vi "16_2.vi"() -> ()   [LabVIEW 2018]
uses:
  <userlib>/_OpenG.lib/array/array.llb/Sort 1D Array (I32)__ogtk.vi
  <userlib>/_OpenG.lib/array/array.llb/Reorder 1D Array2 (I32)__ogtk.vi
  <userlib>/_OpenG.lib/array/array.llb/Reorder 1D Array2 (Variant)__ogtk.vi
panel:
  out "product":dbl
  out "array":i32[](array[numeric])
  out "Array 6":string[](array[string])
  out "Array 2":cluster{string[]}[](array[cluster])
  out "Array 3":i32[](array[numeric])
  out "your ticket":string
  out "nearby tickets":string[](array[string])
  out "first subarray":string[](array[string])
  in  "Input":string
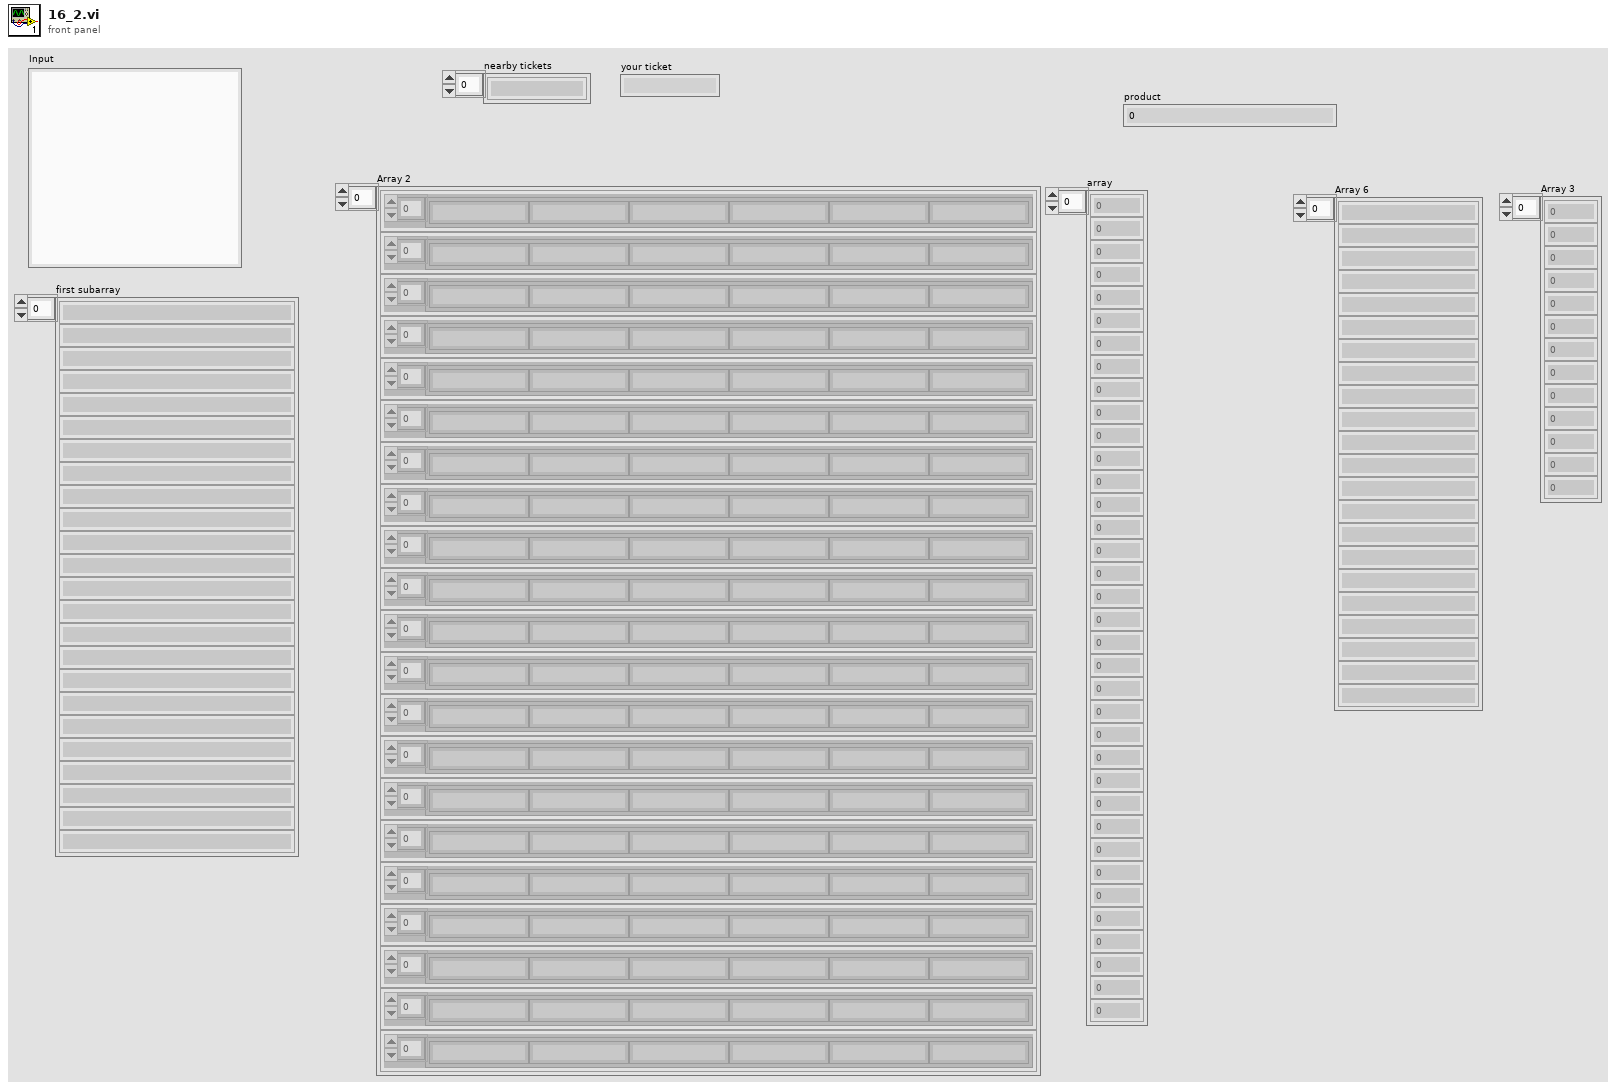
[diagram p1: front panel]
types:
  T1 = cluster{"Min1":i32, "Max1":i32, "Min2":i32, "Max2":i32, "Field":string}
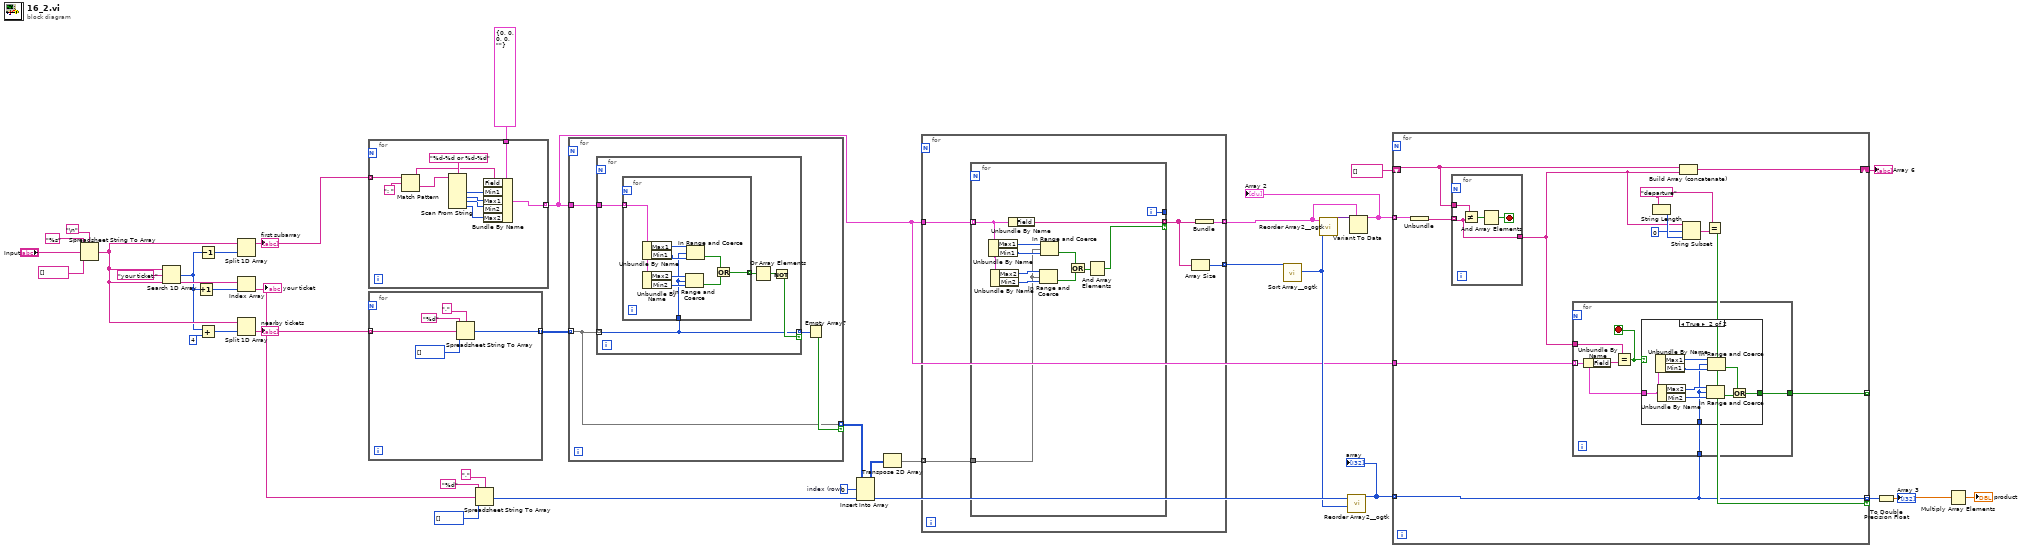
[diagram p0: block diagram]
diagram:
  w19 = 0  # index (row)
  n1 = Spreadsheet String To Array(delimiter (Tab)="\n", format string="%s", spreadsheet string="Input", array type (2D Dbl)=string[] []) -> (array=w29:string[])
  n2 = Search 1D Array(1D array=w29, element="your ticket:") -> (index of element=w27:i32)  [unwired: 1 in]
  n3 = Increment(x=w27) -> (x+1=w30:i32)
  n4 = Decrement(x=w27) -> (x-1=w31:i32)
  n5 = Add(x=w27, y=4) -> (x+y=w28:i32)
  n6 = Split 1D Array(array=w29, index=w31) -> (first subarray=w25:string[])  [unwired: 1 out]
  "first subarray" <- w25
  n7 = Index Array(array=w29, index=w30) -> (element=w20:string)
  "your ticket" <- w20
  n8 = Split 1D Array(array=w29, index=w28) -> (second subarray=w17:string[])  [unwired: 1 out]
  "nearby tickets" <- w17
  n9 = for {
    tunnel: w25 -> [w47] mode=indexing
    tunnel: T1 {"Min1"=0, "Max1"=0, "Min2"=0, "Max2"=0, "Field"=""} -> [w43]
    tunnel: [w38] -> w3 mode=indexing
    n10 = Match Pattern(string=w47, regular expression=": ") -> (before substring=w37:string, after substring=w45:string)  [unwired: 1 in, 2 out]
    n11 = Scan From String(format string="%d-%d or %d-%d", input string=w45) -> (output 1=w42:i32, output 2=w41:i32, output 3=w40:i32, output 4=w39:i32)  [unwired: 6 in, 3 out]
    n12 = Bundle By Name(cluster=w43, "Field"=w37, "Min1"=w42, "Max1"=w41, "Min2"=w40, "Max2"=w39) -> (w38:T1)
  }
  n13 = for {
    tunnel: w17 -> [w49] mode=indexing
    tunnel: [w48] -> w16 mode=indexing
    n14 = Spreadsheet String To Array(delimiter (Tab)=",", format string="%d", spreadsheet string=w49, array type (2D Dbl)=i32[] []) -> (array=w48:i32[])
  }
  n15 = Spreadsheet String To Array(delimiter (Tab)=",", format string="%d", spreadsheet string=w20, array type (2D Dbl)=i32[] []) -> (array=w8:i32[])
  n16 = for {
    tunnel: w16 -> [w53] mode=indexing
    tunnel: w3 -> [w56]
    tunnel: [w53] -> w18 mode=indexing if=w54
    n17 = for {
      tunnel: w53 -> [w57] mode=indexing
      tunnel: w56 -> [w61]
      tunnel: [w57] -> w55 mode=indexing if=w58
      n18 = for {
        tunnel: w61 -> [w66] mode=indexing
        tunnel: w57 -> [w63]
        tunnel: [w62] -> w60 mode=indexing
        n19 = Unbundle By Name(w66) -> ("Max1"=w70:i32, "Min1"=w69:i32)
        n20 = Unbundle By Name(w66) -> ("Max2"=w68:i32, "Min2"=w67:i32)
        n21 = In Range and Coerce(upper limit=w68, x=w63, lower limit=w67) -> (In Range?=w65:bool)  [unwired: 1 out]
        n22 = In Range and Coerce(upper limit=w70, x=w63, lower limit=w69) -> (In Range?=w64:bool)  [unwired: 1 out]
        n23 = Or(x=w64, y=w65) -> (x .or. y?=w62:bool)
      }
      n24 = Or Array Elements(Boolean array=w60) -> (logical OR=w59:bool)
      n25 = Not(x=w59) -> (.not. x?=w58:bool)
    }
    n26 = Empty Array?(array=w55) -> (empty?=w54:bool)
  }
  n27 = Insert Into Array(array=w18, index (row)=w19, new element=w8) -> (w15:i32[][])  [unwired: 1 in]
  n28 = Transpose 2D Array(2D array=w15) -> (transposed array=w14:i32[][])
  n29 = for {
    tunnel: w14 -> [w75] mode=indexing
    tunnel: w3 -> [w74]
    tunnel: [w73] -> w10 mode=indexing
    tunnel: [w71] -> w12 mode=indexing
    n30 = for {
      tunnel: w75 -> [w81]
      tunnel: w74 -> [w79] mode=indexing
      tunnel: [w78] -> w72 mode=indexing if=w76
      tunnel: [w77] -> _
      i -> [w77]
      n31 = Unbundle By Name(w79) -> ("Max1"=w85:i32, "Min1"=w84:i32)
      n32 = Unbundle By Name(w79) -> ("Max2"=w83:i32, "Min2"=w82:i32)
      n33 = Unbundle By Name(w79) -> ("Field"=w78:string)
      n34 = In Range and Coerce(upper limit=w83, x=w81, lower limit=w82) -> (In Range?=w86:bool[])  [unwired: 1 out]
      n35 = In Range and Coerce(upper limit=w85, x=w81, lower limit=w84) -> (In Range?=w87:bool[])  [unwired: 1 out]
      n36 = Or(x=w87, y=w86) -> (x .or. y?=w80:bool[])
      n37 = And Array Elements(Boolean array=w80) -> (logical AND=w76:bool)
    }
    n38 = Array Size(array=w72) -> (size(s)=w71:i32)
    n39 = Bundle(w72) -> (w73:cluster{string[]})  [unwired: 1 in]
  }
  n40 = call-poly <userlib>:"Sort Array__ogtk.vi"("Array in"=w12) -> ("Sorted Pointers"=w7:i32[])  [unwired: 9 in, 1 out]
  n41 = call-poly <userlib>:"Reorder Array2__ogtk.vi"("indices"=w7, "array"=w10) -> ("reordered array"=w11:variant[])  [unwired: 9 in]
  n42 = call-poly <userlib>:"Reorder Array2__ogtk.vi"("indices"=w7, "array"=w8) -> ("reordered array"=w4:i32[])  [unwired: 9 in]
  "array" <- w4
  n43 = Variant To Data(type=w10, Variant=w11) -> (data=w5:cluster{string[]}[])  [unwired: 1 in, 1 out]
  "Array 2" <- w5
  n44 = for {
    tunnel: w5 -> [w95] mode=indexing
    tunnel: [w89] -> w13 mode=indexing if=w96
    shift-right: [w92] -> w6
    shift-left: string[] [] -> [w93]
    tunnel: w4 -> [w89] mode=indexing
    tunnel: w3 -> [w91]
    tunnel: [w88] -> _ mode=indexing
    w97 = "departure"
    n45 = Unbundle(w95) -> (w94:string[])
    n46 = for {
      tunnel: w94 -> [w117] mode=indexing
      tunnel: w93 -> [w119]
      tunnel: [w117] -> w90
      stop <- w116 stop-if-true
      n47 = Not Equal?(x=w119, y=w117) -> (x != y?=w118:bool[])
      n48 = And Array Elements(Boolean array=w118) -> (logical AND=w116:bool)
    }
    n49 = for {
      tunnel: w91 -> [w104] mode=indexing
      tunnel: w90 -> [w105]
      tunnel: w89 -> [w103]
      tunnel: [w101] -> w88
      stop <- w102 stop-if-true
      n50 = Unbundle By Name(w104) -> ("Field"=w106:string)
      n51 = Equal?(x=w105, y=w106) -> (x = y?=w102:bool)
      n52 = case shown="True" w102 {
        tunnel: w104 -> [_ w111]
        tunnel: w103 -> [_ w110]
        tunnel: [_ w107] -> w101
        frame False {
        }
        frame True {
          n53 = Unbundle By Name(w111) -> ("Max1"=w112:i32, "Min1"=w113:i32)
          n54 = Unbundle By Name(w111) -> ("Max2"=w114:i32, "Min2"=w115:i32)
          n55 = In Range and Coerce(upper limit=w114, x=w110, lower limit=w115) -> (In Range?=w109:bool)  [unwired: 1 out]
          n56 = In Range and Coerce(upper limit=w112, x=w110, lower limit=w113) -> (In Range?=w108:bool)  [unwired: 1 out]
          n57 = Or(x=w108, y=w109) -> (x .or. y?=w107:bool)
        }
      }
    }
    n58 = String Length(string=w97) -> (length=w100:i32)
    n59 = Build Array (concatenate)(w93, w90) -> (w92:string[])
    n60 = String Subset(string=w90, offset (0)=0, length (rest)=w100) -> (substring=w98:string)
    n61 = Equal?(x=w97, y=w98) -> (x = y?=w96:bool)
  }
  "Array 6" <- w6
  n62 = To Double Precision Float(number=w13) -> (double precision float=w2:dbl[])
  "Array 3" <- w2
  n63 = Multiply Array Elements(1:w2) -> (0:→"product":dbl)
